vi "Aqusition (SubVI).vi"(0 "Video mode":u32, 5 "Stop (F)":bool, 7 "error in":errorcluster) -> (20 "Image Out":T1(plugin-control), 21 "All Image Buffers Out":T1[](array[typedef]), 26 "Stopped":bool, 27 "error out":errorcluster)   [LabVIEW 2017]
doc: "Creates, and edits acquisitions using the NI Vision Acquisition Express VI.\n\nThe NI Vision Acquisition Wizard is launched by placing the Express VI on the block diagram. Select an acquisition source and configure an acquisition using NI-IMAQ, NI-IMAQdx, or simulate an acquisition by reading an AVI or image files from a folder. After an acquisition is configured, select controls and indicators to be able to programmatically set in LabVIEW. Double-click the Vision Acquisition Express VI to edit the acquisition.\n\nNote: Any images created by the Express VI need to be disposed after use. Use the IMAQ Dispose.vi to cleanup the images output by the Express VI when they are no longer needed."
uses:
  <vilib>/vision/Image Controls.llb/IMAQ Image.ctl
  <vilib>/vision/driver/IMAQdx.llb/IMAQdx Acquisition Mode.ctl
  <vilib>/vision/driver/NI_Vision_Acquisition_Software.lvlib
  <resource>/objmgr/imaqdx.rc
panel:
  # "0 - 640x480"
  # "5 - 1280x720"
  # "30 - 320x240"
  # "35 - 800x600"
  # "40 - 176x144"
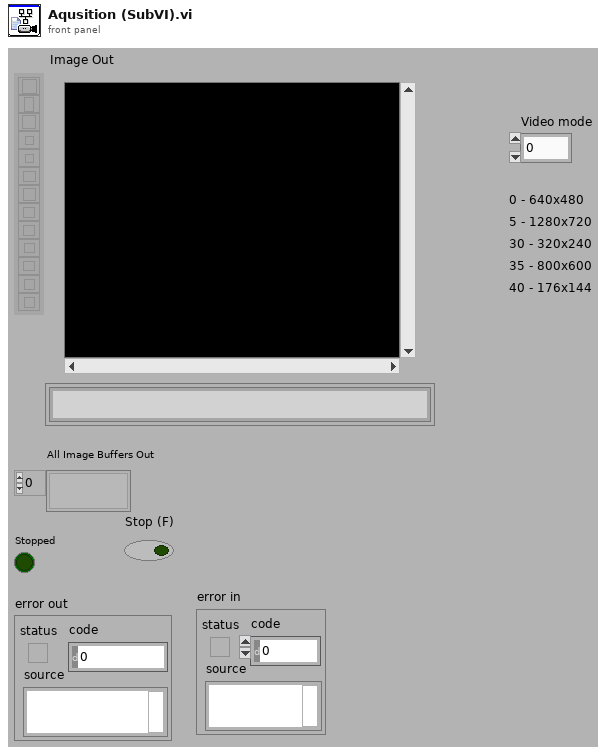
[diagram p1: front panel]
types:
  T1 = typedef "IMAQ Image.ctl" = refnum<image>
  T2 = typedef "NI_Vision_Acquisition_Software.lvlib/IMAQdx Acquisition Mode.ctl" = enum32{"One Shot", "Continuous"}
  T3 = typedef "IMAQdx.ctl" = refnum<k21>
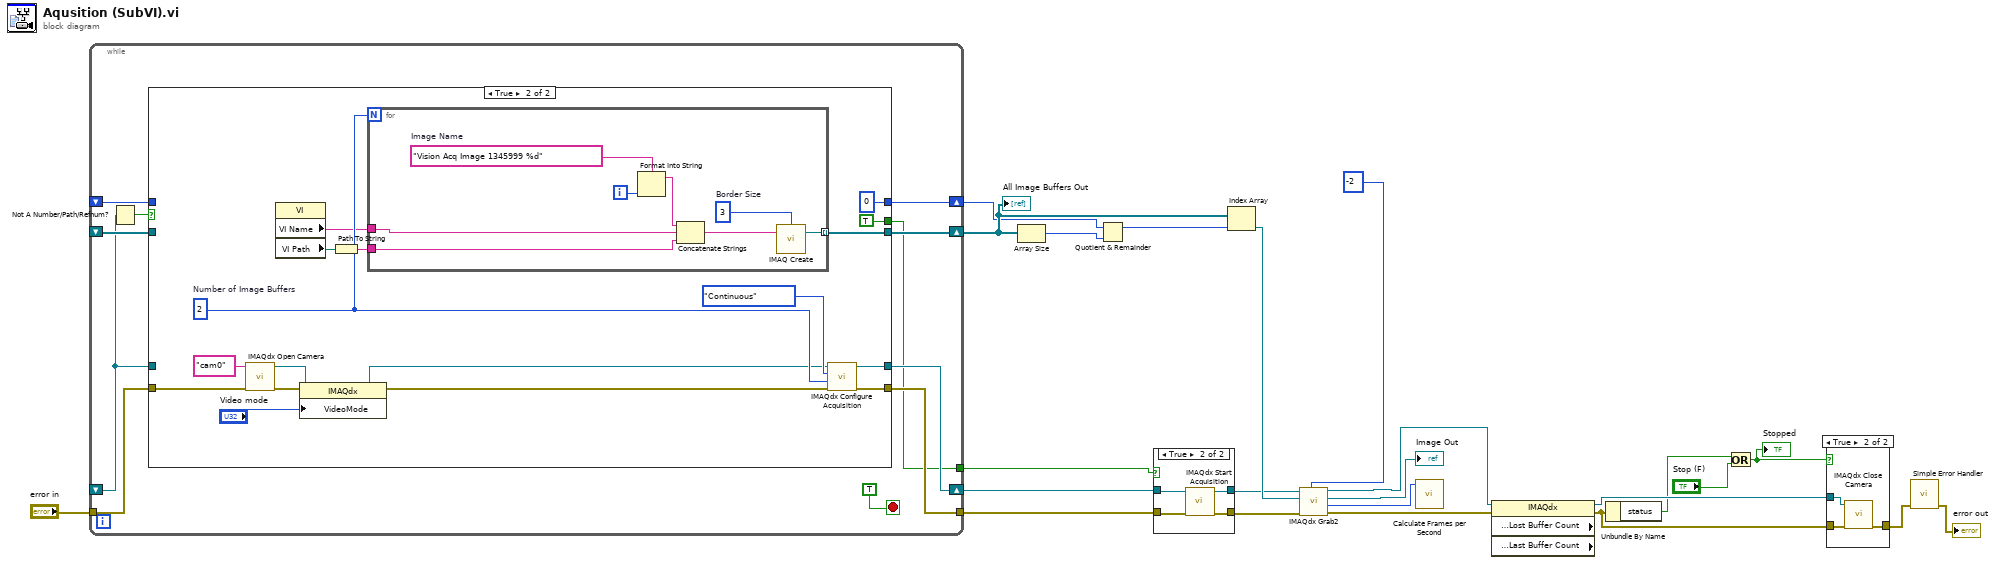
[diagram p0: block diagram]
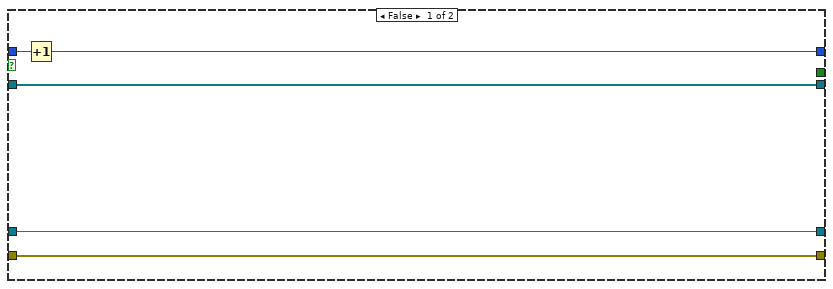
[diagram p4: hidden frame]
diagram:
  n1 = while {
    shift-right: [w34] -> w9
    shift-left: _ -> [w27]
    tunnel: [w33] -> w10
    shift-right: [w31] -> w20
    shift-left: _ -> [w30]
    shift-right: [w29] -> w17
    shift-left: _ -> [w28]
    tunnel: [w25] -> w12
    tunnel: "error in" -> [w24]
    stop <- TRUE stop-if-true
    n2 = Not A Number/Path/Refnum?(number/path/refnum=w27) -> (NaN/Path/Refnum?=w26:bool)
    n3 = case shown="True" w26 {
      tunnel: [w39 w53] -> w34
      tunnel: w27 -> [w39 _]
      tunnel: [w38 w52] -> w33
      tunnel: w24 -> [w38 w55]
      tunnel: [w37 w51] -> w31
      tunnel: w30 -> [w37 _]
      tunnel: [w35 0] -> w29
      tunnel: w28 -> [w36 _]
      tunnel: [_ TRUE] -> w25
      frame False {
        n4 = Increment(x=w36) -> (x+1=w35:i32)
      }
      frame True {
        w50 = u32 2  # Number of Image Buffers
        n5 = call <vilib>:"IMAQdx Open Camera.vi"("error in"=w55, "Session In"="cam0" ("Interface Name")) -> ("error out"=w41:errorcluster, "Session Out"=w43:T3)  [unwired: 1 in, 7 out]
        n6 = property class="VI"() -> ("VI Name"=w47:string, "VI Path"=w48:path)  [unwired: 2 in, 2 out]
        n7 = property class="IMAQdx"(reference=w43, "VideoMode"="Video mode") -> (reference out=w42:T3)  [unwired: 1 in, 1 out]
        n8 = Path To String(path=w48) -> (string=w46:string)
        n9 = for "For Loop_template0" {
          N: w50 -> [_]
          tunnel: [w63] -> w51 mode=indexing
          tunnel: w47 -> [w58]
          tunnel: w46 -> [w57]
          i -> [w62]
          w56 = 3  # Border Size
          w61 = "Vision Acq Image 1345999 %d"  # Image Name
          n10 = Format Into String(format string=w61, w62) -> (resulting string=w60:string)  [unwired: 2 in, 1 out]
          n11 = Concatenate Strings(w60, w58, w57) -> (w59:string)
          n12 = call "IMAQ Create"("Border Size"=w56, "Image Name"=w59) -> ("New Image"=w63:T1)  [unwired: 2 in, 2 out]
        }
        n13 = call <vilib>:"IMAQdx Configure Acquisition.vi"("error in"=w41, "Number of Buffers"=w50, "Continuous?"=IMAQdx_Acquisition_Mode."Continuous", "Session In"=w42) -> ("error out"=w52:errorcluster, "Session Out"=w53:T3)  [unwired: 6 out]
      }
    }
  }
  "All Image Buffers Out" <- w20
  n14 = Array Size(array=w20) -> (size(s)=w21:i32)
  n15 = Quotient & Remainder(x=w17, y=w21) -> (x-y*floor(x/y)=w19:i32)  [unwired: 1 out]
  n16 = case shown="True" w12 {
    tunnel: w9 -> [w65 w66]
    tunnel: w10 -> [w64 w67]
    tunnel: [w64 w68] -> w6
    tunnel: [w65 w69] -> w2
    frame False {
    }
    frame True {
      n17 = call <vilib>:"IMAQdx Start Acquisition.vi"("error in"=w67, "Session In"=w66) -> ("error out"=w68:errorcluster, "Session Out"=w69:T3)  [unwired: 8 in]
    }
  }
  n18 = Index Array(array=w20, index=w19) -> (element=w7:T1)
  n19 = call <vilib>:"IMAQdx Grab2.vi"("Timeout (ms)"=-2, "error in"=w6, "Image In"=w7, "Session In"=w2) -> ("error out"=w3:errorcluster, "Buffer Number Out"=w4:u32, "Image Out"=→"Image Out":T1, "Session Out"=w1:T3)  [unwired: 4 in]
  n20 = call <vilib>:"Calculate Frames per Second.vi"("Buffer Number"=w4) -> ()  [unwired: 2 in, 9 out]
  n21 = property class="IMAQdx" props=["Status Information:Lost Buffer Count", "Status Information:Last Buffer Count"](reference=w1, error in=w3) -> (reference out=w16:T3, error out=w18:errorcluster)  [unwired: 2 out]
  n22 = Unbundle By Name(w18) -> ("status"=w13:bool)
  n23 = Or(x=w13, y="Stop (F)") -> (x .or. y?=w14:bool)
  "Stopped" <- w14
  n24 = case "Case Structure_template1" shown="True" w14 {
    tunnel: [w70 w72] -> w23
    tunnel: w18 -> [w70 w73]
    tunnel: w16 -> [_ w71]
    frame False {
    }
    frame True {
      n25 = call <vilib>:"IMAQdx Close Camera.vi"("error in"=w73, "Session In"=w71) -> ("error out"=w72:errorcluster)  [unwired: 9 out]
    }
  }
  n26 = call <vilib>:"Simple Error Handler.vi"("error in (no error)"=w23) -> ("error out"=→"error out":errorcluster)  [unwired: 4 in, 4 out]
